vi "Tastiera Telefono.vi"() -> ()   [LabVIEW 2022 SP3]
panel:
  in  "Boolean 12":bool
  in  "Boolean 11":bool
  in  "Boolean 10":bool
  in  "Boolean 9":bool
  in  "Boolean 8":bool
  in  "Boolean 7":bool
  in  "Boolean 6":bool
  in  "Boolean 5":bool
  in  "Boolean 4":bool
  in  "Boolean 3":bool
  in  "Boolean 2":bool
  in  "Boolean":bool
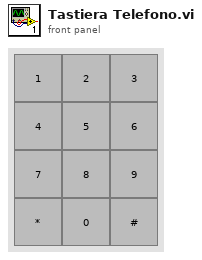
[diagram p1: front panel]
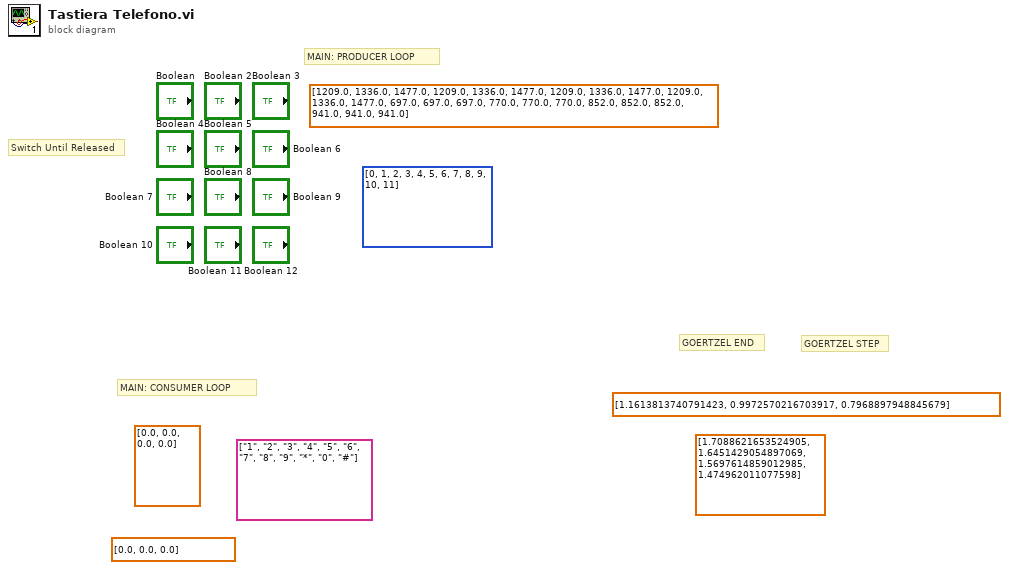
[diagram p0: block diagram]
diagram:
  (unwired) dbl[] [1.7088621653524905, 1.6451429054897069, 1.5697614859012985, 1.474962011077598] ("2cos(L)")
  (unwired) dbl[] [1.1613813740791423, 0.9972570216703917, 0.7968897948845679] ("2cos(H)")
  (unwired) dbl[] [0.0, 0.0, 0.0, 0.0]
  (unwired) dbl[] [0.0, 0.0, 0.0]
  (unwired) string[][] [["1", "2", "3"], ["4", "5", "6"], ["7", "8", "9"], ["*", "0", "#"]]
  (unwired) i16[][] [[0, 1, 2], [3, 4, 5], [6, 7, 8], [9, 10, 11]]
  (unwired) dbl[][] [[1209.0, 1336.0, 1477.0, 1209.0, 1336.0, 1477.0, 1209.0, 1336.0, 1477.0, 1209.0, 1336.0, 1477.0], [697.0, 697.0, 697.0, 770.0, 770.0, 770.0, 852.0, 852.0, 852.0, 941.0, 941.0, 941.0]]
  # "Switch Until Released"
  # "GOERTZEL STEP"
  # "MAIN: CONSUMER LOOP"
  # "MAIN: PRODUCER LOOP"
  # "GOERTZEL END"
